vi "Camera.vi"(10 "Image In":T1, 11 "IMAQ Session In":refnum<k11>) -> (0 "Line Cam Obstacles":cluster{dbl[], dbl[], i32}, 2 "Image (out)":T1, 3 "IMAQ Session Out":refnum<k11>)   [LabVIEW 2011]
uses:
  <vilib>/vision/Image Controls.llb/IMAQ Image.ctl
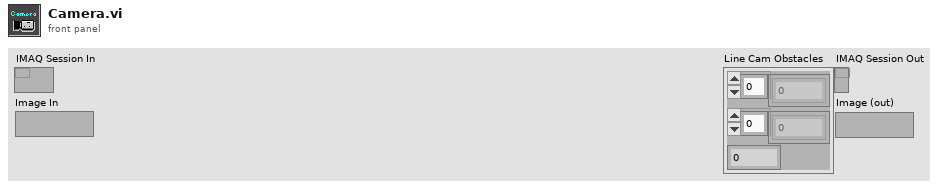
[diagram p1: front panel]
types:
  T1 = typedef "IMAQ Image.ctl" = refnum<image>
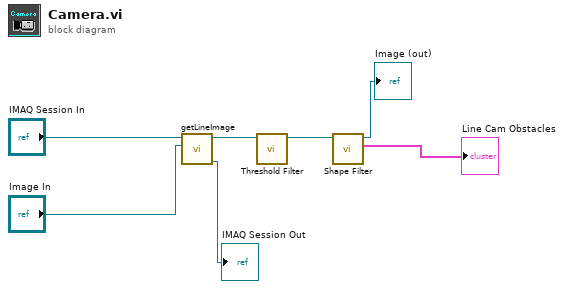
[diagram p0: block diagram]
diagram:
  n1 = call "getLineImage.vi"("Image In"="Image In", "IMAQ Session In"="IMAQ Session In") -> ("IMAQ Session Out"=→"IMAQ Session Out":refnum<k11>, "Image Out"=w7:T1)  [unwired: 8 in]
  n2 = call "Threshold Filter.vi"("Image In"=w7) -> ("Image Out"=w6:T1)  [unwired: 10 in]
  n3 = call "Shape Filter.vi"("Image In"=w6) -> ("Line Cam Obstacles"=→"Line Cam Obstacles":cluster{dbl[], dbl[], i32}, "Image (out)"=→"Image (out)":T1)  [unwired: 9 in]
